vi "MCCMSG Create Object.vi"(8 "error in (no error)":errorcluster, 11 "pnError":i32) -> (0 "error out":errorcluster, 2 "function return":i32, 3 "pnError out":i32)   [LabVIEW 2012, in "MultiClamp 700B Controls.lvlib" / "AxMultiClampMsg.lvlib"]
doc: "AXMCCMSG HMCCMSG WINAPI MCCMSG_CreateObject(int *pnError);"
uses:
  AxMultiClampMsg.lvlib
  AxMultiClampMsg.dll
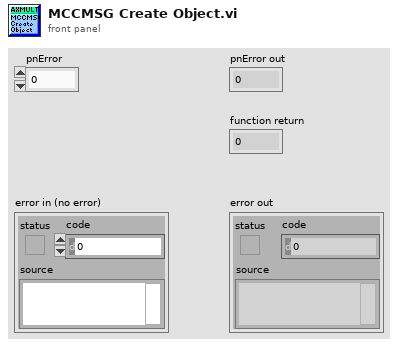
[diagram p1: front panel]
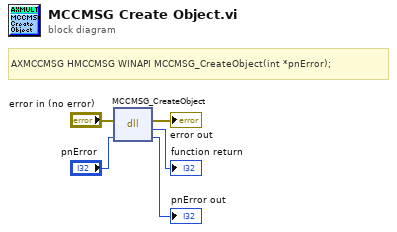
[diagram p0: block diagram]
diagram:
  # "AXMCCMSG HMCCMSG WINAPI MCCMSG_CreateObject(int *pnError);"
  n1 = dll-call lib="C:/Users/Southampton/Desktop/Rita/Multiclamp 700B VIs/AxMultiClampMsg/AxMultiClampMsg.dll" fn="MCCMSG_CreateObject"(error in="error in (no error)", "pnError"="pnError") -> (error out=→"error out":errorcluster, "return type"=→"function return":i32, "pnError"=→"pnError out":i32)  [unwired: 2 in, 1 out]
